vi "Stop Core.vi"(10 "final error code":i32, 11 "Nested in":refnum<class "NXP.lvclass">) -> (3 "Nested out":refnum<class "NXP.lvclass">)   [LabVIEW 2019, in "NXP.lvclass"]
doc: "(<B>Filename</B>: Actor Framework.lvlib:Actor.lvclass:Stop Core.vi)\n\nDefines what the actor does before it stops. Use the <B>final error code</B> input to determine whether the actor shut down in response to an error.\n\nBy default, this method does nothing. A descendant class may override it to define behavior, such as shutting down any processes the actor initiated in its override of the Actor Core method."
uses:
  NXP.lvclass
  Serial Devices/Serial Devices.lvclass
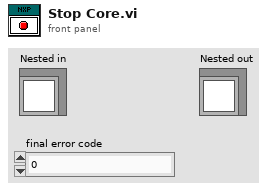
[diagram p1: front panel]
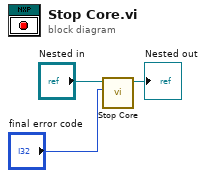
[diagram p0: block diagram]
diagram:
  n1 = call-parent "Stop Core.vi"("final error code"="final error code", "Nested in"="Nested in") -> ("Nested out"=→"Nested out":refnum<class "NXP.lvclass">)  [unwired: 9 in]
